vi "Forlooping shift register.vi"() -> ()   [LabVIEW 2018]
panel:
  out "x+y":dbl
  out "Numeric":i32
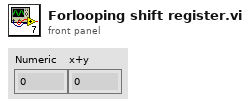
[diagram p1: front panel]
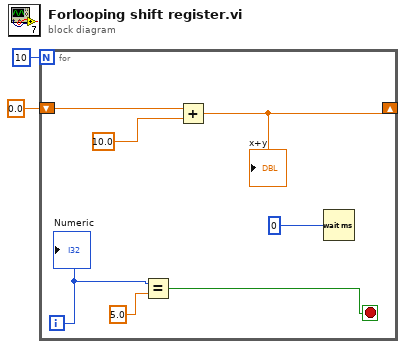
[diagram p0: block diagram]
diagram:
  n1 = for {
    N: 10 -> [_]
    shift-right: [w6] -> _
    shift-left: 0.0 -> [w7]
    i -> [w3]
    stop <- w5 stop-if-true
    n2 = Equal?(x=w3, y=5.0) -> (x = y?=w5:bool)
    n3 = Add(x=w7, y=10.0) -> (x+y=w6:dbl)
    "x+y" <- w6
    n4 = Wait (ms)(milliseconds to wait=0) -> ()  [unwired: 1 out]
    "Numeric" <- w3
  }
